vi "ExSubSetInitCamcascadeorcoolsnap.vi"(2 "Name":string, 3 "overlap mode":bool, 4 "error in (no error)":errorcluster, 5 "Intensifier":bool, 6 "Exposure":dbl min=0.0 step=0.001 format="%.3f", 7 "Camera Handle":u32) -> (0 "error out":errorcluster, 1 "Handles Out":T1)   [LabVIEW 2010]
panel:
  # "ExSubSetInitCam:\nThis sub vi initializes the camera."
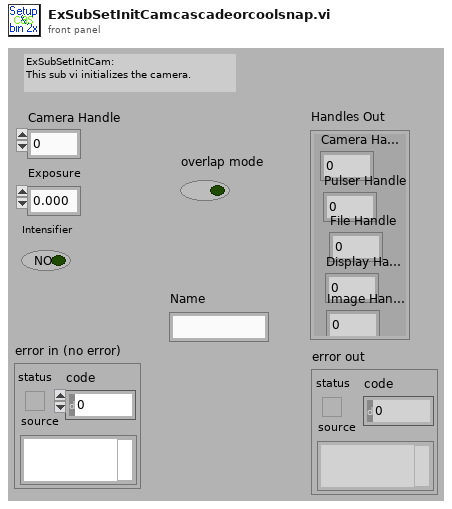
[diagram p1: front panel]
types:
  T1 = cluster{"Camera Handle":u32, "Pulser Handle":u32, "File Handle":u32, "Display Handle":u32, "Image Handle":u32}
  T2 = cluster{"acquire focus mode":u32, "Exposure":dbl, "Number of Images":u32, "Software accumulation":u32}
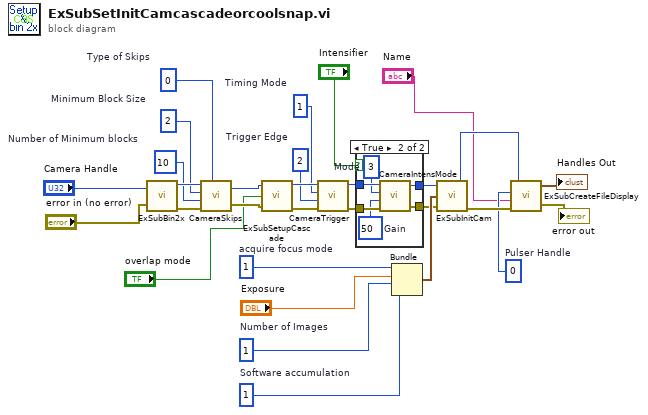
[diagram p0: block diagram]
diagram:
  w13 = u32 0  # Pulser Handle
  w14 = u32 1  # Timing Mode
  w15 = u32 2  # Trigger Edge
  w18 = u32 1  # acquire focus mode
  w17 = u32 1  # Number of Images
  w16 = u32 1  # Software accumulation
  w19 = u32 0  # Type of Skips
  w20 = u32 2  # Minimum Block Size
  w21 = u32 10  # Number of Minimum blocks
  n1 = call "ExSubBin2x.vi"("error in (no error)"="error in (no error)", "Camera Handle"="Camera Handle") -> ("error out"=w22:errorcluster, "Camera Handle"=w23:u32)
  n2 = call <userlib>:"CameraSkips.vi"("Camera Handle"=w23, "Minimum Block Size"=w20, "Number of Minimum blocks"=w21, "error in"=w22, "Type of Skips"=w19) -> ("Camera Handle"=w25:u32, "error out"=w24:errorcluster)
  n3 = call "ExSubSetupCascade.vi"("error in (no error)"=w24, "OverLap Mode"="overlap mode", "Camera Handle"=w25) -> ("error out"=w26:errorcluster, "Camera Handle"=w27:u32)
  n4 = call <userlib>:"CameraTrigger.vi"("error in"=w26, "Trigger Edge"=w15, "Timing Mode"=w14, "Camera Handle"=w27) -> ("error out"=w10:errorcluster, "Camera Handle"=w12:u32)
  n5 = case shown="True" "Intensifier" {
    tunnel: w12 -> [w32 w38]
    tunnel: [w32 w37] -> w11
    tunnel: w10 -> [w31 w36]
    tunnel: [w31 w35] -> w9
    frame False {
    }
    frame True {
      w33 = u32 50  # Gain
      w34 = u32 3  # Mode
      n6 = call <userlib>:"CameraIntensMode.vi"("error in"=w36, "Intensifier Gain"=w33, "Mode"=w34, "Camera Handle"=w38) -> ("error out"=w35:errorcluster, "Camera Handle"=w37:u32)
    }
  }
  n7 = Bundle("acquire focus mode"=w18, "Exposure"="Exposure", "Number of Images"=w17, "Software accumulation"=w16) -> (w29:T2)  [unwired: 1 in]
  n8 = call "ExSubInitCam.vi"("error in (no error)"=w9, "Camera Information"=w29, "Camera Handle"=w11) -> ("error out"=w28:errorcluster, "Camera Handle"=w4:u32)
  n9 = call "ExSubCreateFileDisplay.vi"("error in (no error)"=w28, "File and Display Name"="Name", "Pulser Handle"=w13, "Camera Handle"=w4) -> ("error out"=→"error out":errorcluster, "Handles Out"=→"Handles Out":T1)
